vi "RS_SMBV100A_N_in_SKY_to_SAT_in_DEVICE.vi"(0 "DriverConnect in":T1={"InterfaceType"=enum."VISA", "OpenedSession"="", "InterfaceSettings"={"Interface"=enum."RS232", "EOS 4 read"=enum."LF (\\n)", "EOS 4 write"=enum."LF (\\n)", "TMO, ms"=10000, "Sett"=variant(cluster{"Baud Rate":u32, "Data Bits":u16, "Parity":u16, "Stop Bits":u16, "Flow Control":u16, "Eho":bool} {"Baud Rate"=75, "Data Bits"=0, "Parity"=0, "Stop Bits"=0, "Flow Control"=0, "Eho"=FALSE})}}, 1 "BASEBAND":string, 11 "Error In":errorcluster, 12 "String Value":string) -> (3 "GNSS":string, 4 "DriverConnect out":T1={"InterfaceType"=enum."VISA", "OpenedSession"="", "InterfaceSettings"={"Interface"=enum."RS232", "EOS 4 read"=enum."LF (\\n)", "EOS 4 write"=enum."LF (\\n)", "TMO, ms"=10000, "Sett"=variant(cluster{"Baud Rate":u32, "Data Bits":u16, "Parity":u16, "Stop Bits":u16, "Flow Control":u16, "Eho":bool} {"Baud Rate"=75, "Data Bits"=0, "Parity"=0, "Stop Bits"=0, "Flow Control"=0, "Eho"=FALSE})}}, 13 "SATINSKY_for_DEVICE":dbl, 14 "SAT":dbl, 15 "Error Out":errorcluster)   [LabVIEW 2018]
uses:
  MOKO_LabViewLibrary/MokoLowLevel/MokoLowLovelControl/MLLC_ConnectCluster.ctl
  MOKO_LabViewLibrary/MokoLowLevel/MokoLowLovelControl/MLLC_InterfaceType.ctl
  MOKO_LabViewLibrary/MokoLowLevel/MokoLowLovelControl/MLLC_OpenedSession.ctl
  MOKO_LabViewLibrary/MokoLowLevel/MokoLowLovelControl/MLLC_InterfaceSettings.ctl
  MOKO_LabViewLibrary/MokoLowLevel/MokoLowLovelControl/MLLC_InterfaceKind.ctl
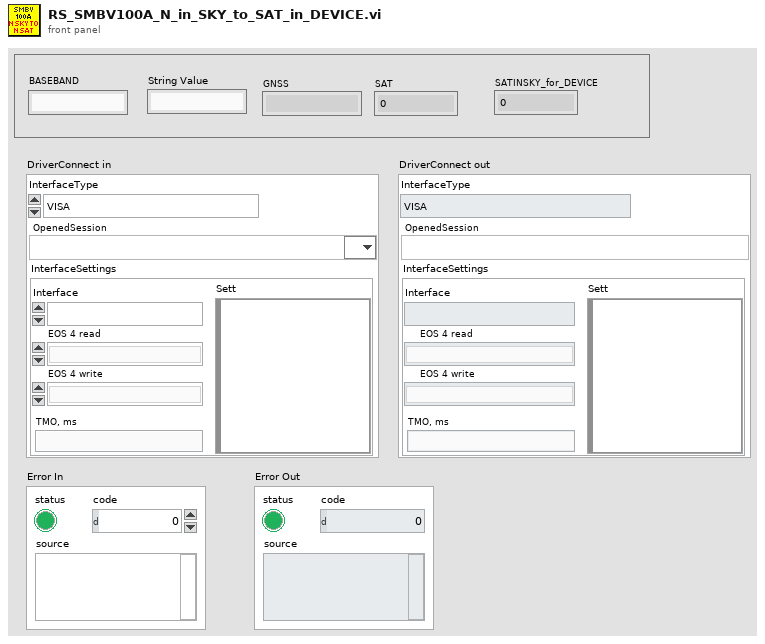
[diagram p1: front panel]
types:
  T1 = typedef "MLLC_ConnectCluster.ctl" = cluster{"InterfaceType":T2, "OpenedSession":T3, "InterfaceSettings":T4}
  T2 = typedef "MLLC_InterfaceType.ctl" = enum16{"VISA", "Prologix USB-GPIB"}
  T3 = typedef "MLLC_OpenedSession.ctl" = refnum<visa-resource-name>
  T4 = typedef "MLLC_InterfaceSettings.ctl" = cluster{"Interface":T5, "EOS 4 read":enum16{"Default (=EOS 4 write)", "CR (\\r)", "LF (\\n)", "None"}, "EOS 4 write":enum16{"CR+LF (\\r\\n)", "CR (\\r)", "LF (\\n)", "None"}, "TMO, ms":i32, "Sett":variant}
  T5 = typedef "MLLC_InterfaceKind.ctl" = enum16{"RS232", "GPIB", "USB", "Ethernet", "another"}
  T6 = typedef "RS_SMBV100A_Parsing Satelite.ctl" = cluster{"Time":dbl[], "Sat":dbl[], "State":dbl[], "NUMBERINSKY":dbl[], "STANDART":string[]}
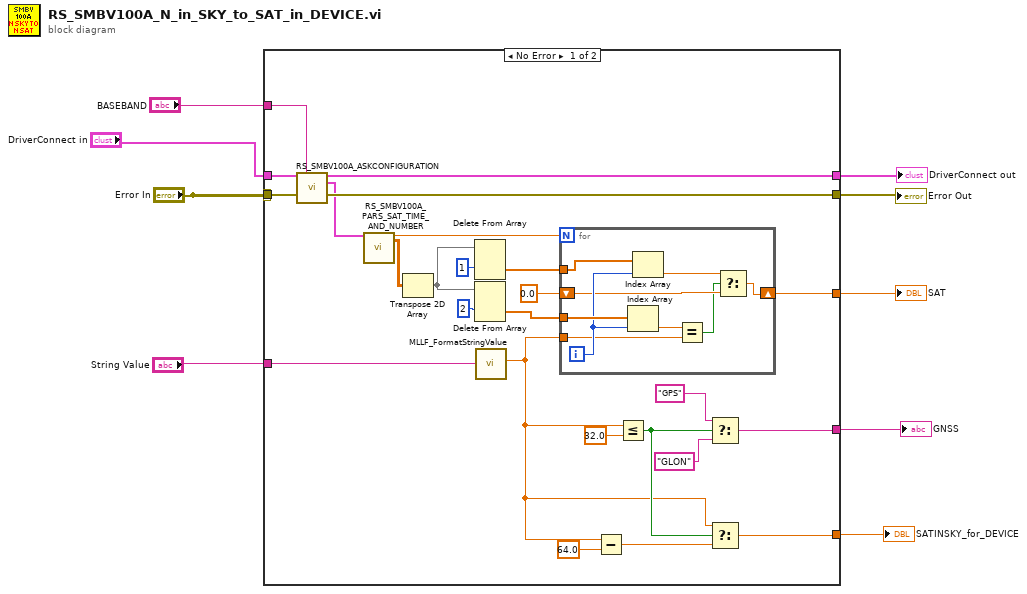
[diagram p0: block diagram]
diagram:
  n1 = case shown="No Error" "Error In" {
    selector: "Error In" -> [_ w44]
    tunnel: [w34 w44] -> w3
    tunnel: "BASEBAND" -> [w27 _]
    tunnel: "DriverConnect in" -> [w26 w45]
    tunnel: "Error In" -> [w25 _]
    tunnel: [w24 w45] -> w1
    tunnel: "String Value" -> [w23 _]
    tunnel: [w22 _] -> w7
    tunnel: [w18 _] -> w6
    tunnel: [w11 _] -> w5
    frame No Error {
      n2 = call "RS_SMBV100A_ASKCONFIGURATION.vi"("DriverConnect in"=w26, "BASEBAND"=w27, "Error In"=w25) -> ("DriverConnect out"=w24:T1, "Parsing Satelite"=w10:T6, "Error Out"=w34:errorcluster)  [unwired: 10 in]
      n3 = call "RS_SMBV100A_PARS_SAT_TIME_AND_NUMBER.vi"("Parsing Satelite"=w10) -> ("OUT GNSS NUMBERACTIVESAT"=w28:dbl, "GNSS 2D SAT"=w17:dbl[][])  [unwired: 13 in, 4 out]
      n4 = Transpose 2D Array(2D array=w17) -> (transposed array=w16:dbl[][])
      n5 = Delete From Array(array=w16, index (row)=1) -> (deleted portion=w30:dbl[])  [unwired: 2 in, 1 out]
      n6 = Delete From Array(array=w16, index (row)=2) -> (deleted portion=w31:dbl[])  [unwired: 2 in, 1 out]
      n7 = call "MLLF_FormatStringValue.vi"("String Value"=w23) -> ("number"=w14:dbl)  [unwired: 8 in, 2 out]
      n8 = for {
        N: w28 -> [_]
        tunnel: w31 -> [w43]
        tunnel: w30 -> [w41]
        shift-right: [w36] -> w22
        shift-left: 0.0 ("y") -> [w38]
        tunnel: w14 -> [w35]
        i -> [w40]
        n9 = Index Array(array=w43, index=w40) -> (element=w42:dbl)
        n10 = Index Array(array=w41, index=w40) -> (element=w39:dbl)
        n11 = Equal?(x=w42, y=w35) -> (x = y?=w37:bool)
        n12 = Select(t=w39, s=w37, f=w38) -> (s? t:f=w36:dbl)
      }
      n13 = Subtract(x=w14, y=64.0) -> (x-y=w12:dbl)
      n14 = Less Or Equal?(x=w14, y=32.0) -> (x <= y?=w15:bool)
      n15 = Select(t="GPS", s=w15, f="GLON") -> (s? t:f=w18:string)
      n16 = Select(t=w14, s=w15, f=w12) -> (s? t:f=w11:dbl)
    }
    frame Error {
    }
  }
  "SAT" <- w7
  "GNSS" <- w6
  "SATINSKY_for_DEVICE" <- w5
  "Error Out" <- w3
  "DriverConnect out" <- w1
